vi "CRYCalc Constant Wave Unit.vi"(6 "B_axis mode":u16(slide) scale=0.0..2.0, 7 "A_axis mode":u16(slide) scale=0.0..2.0, 8 "Value in":T2={"Name"="", "Curve"=[], "X data"=1, "Y data"=1, "Z data"=1, "X axis"=0, "Y axis"=1, "Z axis"=1, "X unit"="Hz", "Y unit"="", "Z unit"="deg.", "X dB ref"=1.0, "Y dB ref"=1.0, "Z dB ref"=1.0, "single val"=FALSE, "protected"=FALSE, "display X"=TRUE, "display Y"=TRUE, "display Z"=TRUE, "Test Info"="", "Step No."=0, "Plot Settings"={"Color"=0, "Interpolation"=0, "Point Style"=0, "Line Style"=0, "Point Color"=0, "Line Width"=0, "Bar Plot Style"=0, "Fill To"=0}, "AutoProtect"=FALSE} {"Z data" items=["dB", "Lin"]; "X data" items=["dB", "Lin"]; "Y data" items=["dB", "Lin"]; "Z dB ref" format="%.1f"; "Z axis" items=["Log", "Lin"]; "X dB ref" format="%.1f"; "X axis" items=["Log", "Lin"]; "Y axis" items=["Log", "Lin"]; "Y dB ref" format="%.1f"; "Curve"."z" format="%.2f"; "Curve"."y" format="%.2f"; "Curve"."x" format="%.2f"}, 9 "Work in":u16(slide), 10 "Operator":u16(ring) items=["+", "--", "x", "/"], 11 "Wave in":T1={"Waveform"={"X0"=0.0, "dX"=0.0, "Y"=[]}, "X data"=1, "Y data"=1, "Y axis"=1, "X unit"="s", "Y unit"="V", "Y dB ref"=1.0, "display Y"=TRUE, "display X"=TRUE, "Overload?"=FALSE, "Test Info"="", "Step No."=0, "Name"="", "protected"=FALSE, "Sqc history"=[], "Signal Channel ID"=0, "Plot Settings"={"Color"=0, "Interpolation"=0, "Point Style"=0, "Line Style"=0, "Point Color"=0, "Line Width"=0, "Bar Plot Style"=0, "Fill To"=0}, "AutoProtect"=FALSE} {"Y dB ref" format="%.1f"; "Y axis" items=["Log", "Lin"]; "Y data" items=["dB", "Lin"]; "X data" items=["dB", "Lin"]}) -> (2 "Wave out":T1={"Waveform"={"X0"=0.0, "dX"=0.0, "Y"=[]}, "X data"=1, "Y data"=1, "Y axis"=1, "X unit"="s", "Y unit"="V", "Y dB ref"=1.0, "display Y"=TRUE, "display X"=TRUE, "Overload?"=FALSE, "Test Info"="", "Step No."=0, "Name"="", "protected"=FALSE, "Sqc history"=[], "Signal Channel ID"=0, "Plot Settings"={"Color"=0, "Interpolation"=0, "Point Style"=0, "Line Style"=0, "Point Color"=0, "Line Width"=0, "Bar Plot Style"=0, "Fill To"=0}, "AutoProtect"=FALSE} {"Y dB ref" format="%.1f"; "Y axis" items=["Log", "Lin"]; "Y data" items=["dB", "Lin"]; "X data" items=["dB", "Lin"]})   [LabVIEW 2013]
uses:
  Typedef Control/CRYWaveform Cluster.ctl
  Typedef Control/CRYData Cluster.ctl
  CRYPost Processing Global.vi
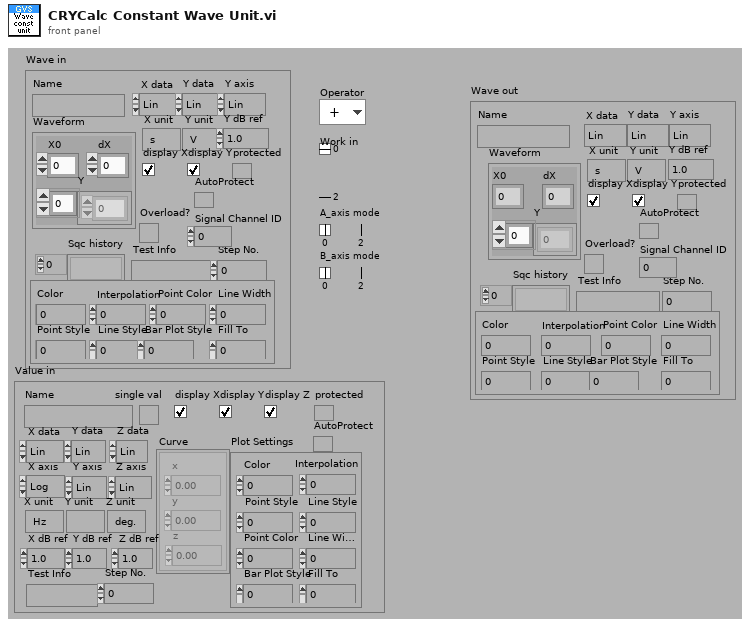
[diagram p1: front panel]
types:
  T1 = typedef "CRYWaveform Cluster.ctl" = cluster{"Waveform":cluster{"X0":dbl, "dX":dbl, "Y":sgl[]}, "X data":u16, "Y data":u16, "Y axis":u16, "X unit":string, "Y unit":string, "Y dB ref":dbl, "display Y":bool, "display X":bool, "Overload?":bool, "Test Info":string, "Step No.":i32, "Name":string, "protected":bool, "Sqc history":string[], "Signal Channel ID":i32, "Plot Settings":cluster{"Color":u32, "Interpolation":u8, "Point Style":u8, "Line Style":u8, "Point Color":u32, "Line Width":u8, "Bar Plot Style":u8, "Fill To":i16}, "AutoProtect":bool}
  T2 = typedef "CRYData Cluster.ctl" = cluster{"Name":string, "Curve":cluster{"x":dbl, "y":dbl, "z":dbl}[], "X data":u16, "Y data":u16, "Z data":u16, "X axis":u16, "Y axis":u16, "Z axis":u16, "X unit":string, "Y unit":string, "Z unit":string, "X dB ref":dbl, "Y dB ref":dbl, "Z dB ref":dbl, "single val":bool, "protected":bool, "display X":bool, "display Y":bool, "display Z":bool, "Test Info":string, "Step No.":i32, "Plot Settings":cluster{"Color":u32, "Interpolation":u8, "Point Style":u8, "Line Style":u8, "Point Color":u32, "Line Width":u8, "Bar Plot Style":u8, "Fill To":i16}, "AutoProtect":bool}
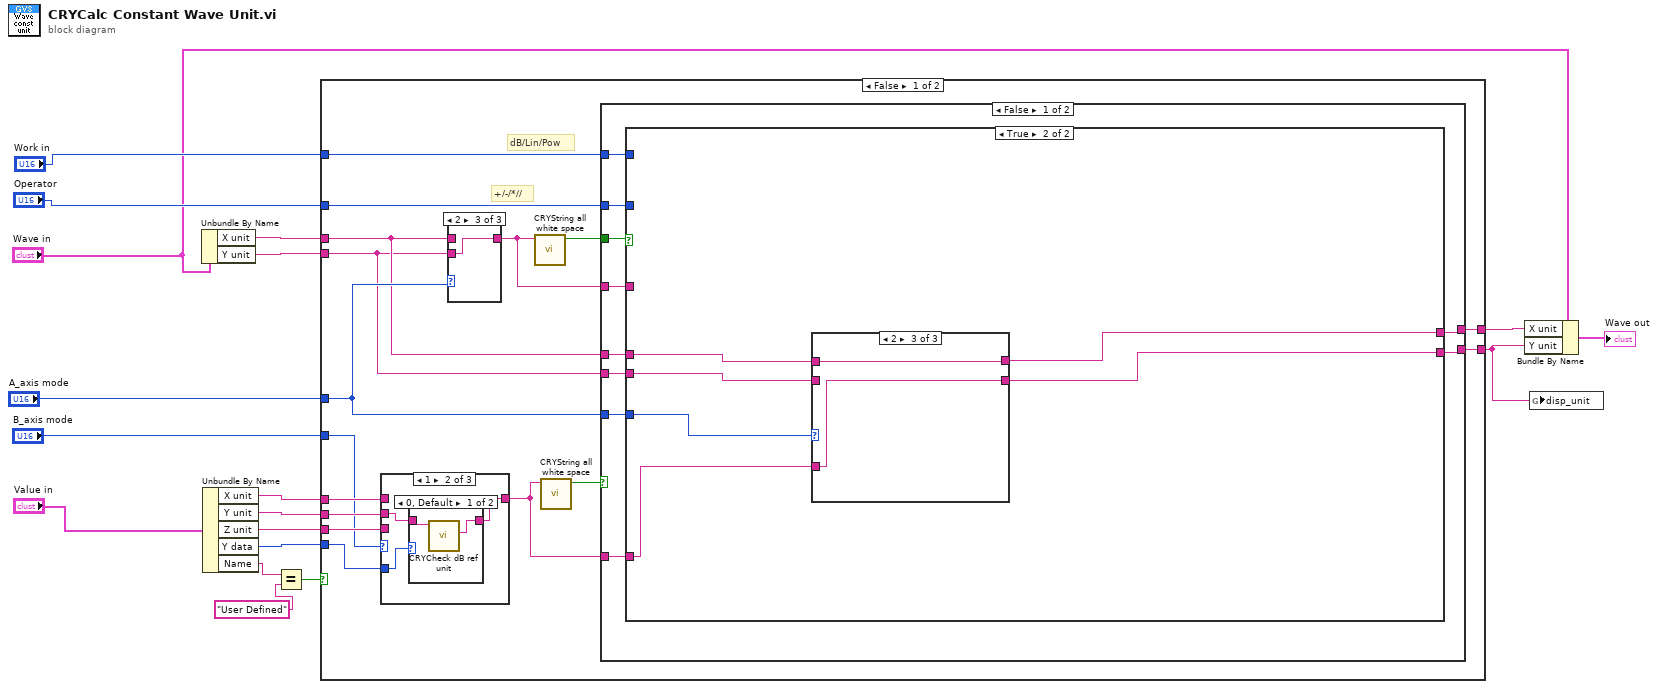
[diagram p0: block diagram]
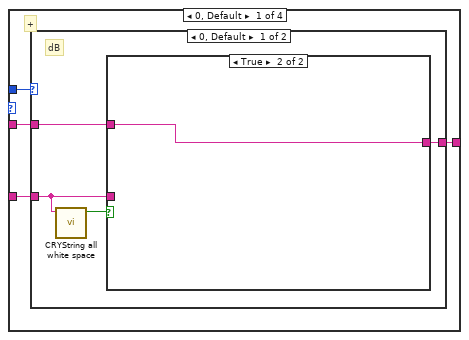
[diagram p7: hidden frame]
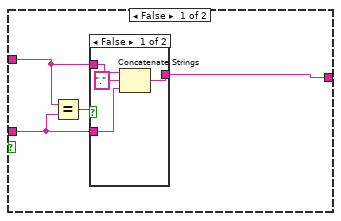
[diagram p8: hidden frame]
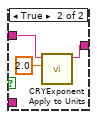
[diagram p9: hidden frame]
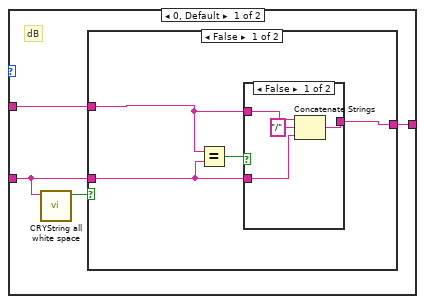
[diagram p11: hidden frame]
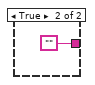
[diagram p12: hidden frame]
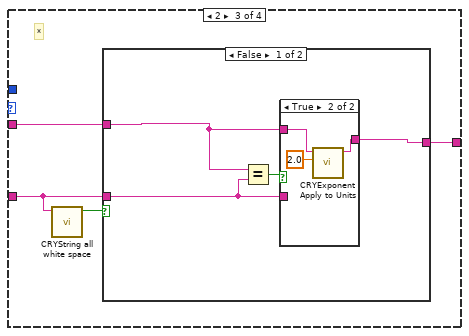
[diagram p14: hidden frame]
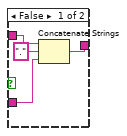
[diagram p15: hidden frame]
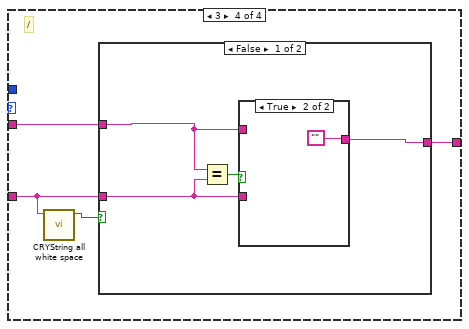
[diagram p17: hidden frame]
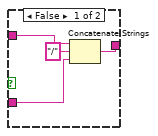
[diagram p18: hidden frame]
diagram:
  n1 = Unbundle By Name("Wave in") -> ("X unit"=w17:string, "Y unit"=w8:string)
  n2 = Unbundle By Name("Value in") -> ("X unit"=w16:string, "Y unit"=w18:string, "Z unit"=w15:string, "Y data"=w10:u16, "Name"=w13:string)
  n3 = Equal?(x=w13, y="User Defined") -> (x = y?=w11:bool)
  n4 = case shown="False" w11 {
    tunnel: w8 -> [w31 w162]
    tunnel: "Operator" -> [w25 _]
    tunnel: "Work in" -> [w26 _]
    tunnel: w18 -> [w23 _]
    tunnel: "A_axis mode" -> [w33 _]
    tunnel: "B_axis mode" -> [w21 _]
    tunnel: w17 -> [w32 w163]
    tunnel: w16 -> [w24 _]
    tunnel: w15 -> [w22 _]
    tunnel: [w29 w163] -> w12
    tunnel: [w30 w162] -> w9
    tunnel: w10 -> [w19 _]
    frame False {
      # "+/-/*//"
      # "dB/Lin/Pow"
      n5 = case shown="1" w21 {
        tunnel: w24 -> [w35 _ _]
        tunnel: w23 -> [_ w37 _]
        tunnel: w22 -> [_ _ w42]
        tunnel: [w35 w36 w42] -> w20
        tunnel: w19 -> [_ w38 _]
        frame 0, Default {
        }
        frame 1 {
          n6 = case shown="0, Default" w38 {
            tunnel: w37 -> [w40 w41]
            tunnel: [w39 w41] -> w36
            frame 0, Default {
              n7 = call "CRYCheck dB ref unit.vi"("Unit in"=w40) -> ("Lin unit out"=w39:string)  [unwired: 1 in, 9 out]
            }
            frame 1 {
            }
          }
        }
        frame 2 {
        }
      }
      n8 = case shown="2" w33 {
        tunnel: w32 -> [w159 w160 _]
        tunnel: w31 -> [_ _ w161]
        tunnel: [w159 w160 w161] -> w27
        frame 0, Default {
        }
        frame 1 {
        }
        frame 2 {
        }
      }
      n9 = call "CRYString all white space.vi"("String"=w27) -> ("Nothing but white space?"=w28:bool)  [unwired: 10 in]
      n10 = call "CRYString all white space.vi"("String"=w20) -> ("Nothing but white space?"=w34:bool)  [unwired: 10 in]
      n11 = case shown="False" w34 {
        tunnel: w33 -> [w52 _]
        tunnel: w32 -> [w49 w158]
        tunnel: w31 -> [w51 w157]
        tunnel: [w50 w157] -> w30
        tunnel: [w47 w158] -> w29
        tunnel: w20 -> [w48 _]
        tunnel: w28 -> [w46 _]
        tunnel: w27 -> [w45 _]
        tunnel: w26 -> [w44 _]
        tunnel: w25 -> [w43 _]
        frame False {
          n12 = case shown="True" w46 {
            tunnel: w52 -> [w53 w150]
            tunnel: w51 -> [w57 w149]
            tunnel: [w55 w148] -> w50
            tunnel: w49 -> [w58 w147]
            tunnel: w48 -> [w59 w146]
            tunnel: [w54 w145] -> w47
            tunnel: w45 -> [w60 _]
            tunnel: w44 -> [w61 _]
            tunnel: w43 -> [w62 _]
            frame False {
              n13 = case shown="2" w53 {
                tunnel: w62 -> [_ w68]
                tunnel: w61 -> [_ w67]
                tunnel: w60 -> [w63 w66]
                tunnel: w59 -> [_ w65]
                tunnel: [w63 w64] -> w56
                frame 0, 1, Default {
                }
                frame 2 {
                  n14 = case shown="1" w68 {
                    tunnel: w67 -> [w72 w93 _ _]
                    tunnel: w66 -> [w71 w92 w112 w128]
                    tunnel: w65 -> [w70 w91 w110 w126]
                    tunnel: [w69 w90 w111 w127] -> w64
                    frame 0, Default {
                      # "+"
                      n15 = case shown="0, Default" w72 {
                        tunnel: w71 -> [w76 w89]
                        tunnel: w70 -> [w74 _]
                        tunnel: [w75 w89] -> w69
                        frame 0, Default {
                          # "dB"
                          n16 = call "CRYString all white space.vi"("String"=w74) -> ("Nothing but white space?"=w73:bool)  [unwired: 10 in]
                          n17 = case shown="True" w73 {
                            tunnel: w76 -> [w80 w88]
                            tunnel: [w79 w88] -> w75
                            tunnel: w74 -> [w78 _]
                            frame False {
                              n18 = Equal?(x=w80, y=w78) -> (x = y?=w77:bool)
                              n19 = case shown="False" w77 {
                                tunnel: w80 -> [w83 w86]
                                tunnel: [w84 w85] -> w79
                                tunnel: w78 -> [w81 _]
                                frame False {
                                n20 = Concatenate Strings(w83, "." ("string"), w81) -> (w84:string)
                                }
                                frame True {
                                n21 = call "CRYExponent Apply to Units.vi"("Exponent to apply"=2.0, "Unit in"=w86) -> ("Unit out"=w85:string)  [unwired: 9 out]
                                }
                              }
                            }
                            frame True {
                            }
                          }
                        }
                        frame 1, 2 {
                          # "Lin,Pow"
                        }
                      }
                    }
                    frame 1 {
                      # "-"
                      n22 = case shown="1, 2" w93 {
                        tunnel: w92 -> [w97 w108]
                        tunnel: w91 -> [w95 _]
                        tunnel: [w96 w108] -> w90
                        frame 0, Default {
                          # "dB"
                          n23 = call "CRYString all white space.vi"("String"=w95) -> ("Nothing but white space?"=w94:bool)  [unwired: 10 in]
                          n24 = case shown="False" w94 {
                            tunnel: w97 -> [w101 w107]
                            tunnel: [w100 w107] -> w96
                            tunnel: w95 -> [w99 _]
                            frame False {
                              n25 = Equal?(x=w101, y=w99) -> (x = y?=w98:bool)
                              n26 = case shown="False" w98 {
                                tunnel: w101 -> [w104 _]
                                tunnel: [w105 ""] -> w100
                                tunnel: w99 -> [w102 _]
                                frame False {
                                n27 = Concatenate Strings(w104, "/" ("string"), w102) -> (w105:string)
                                }
                                frame True {
                                }
                              }
                            }
                            frame True {
                            }
                          }
                        }
                        frame 1, 2 {
                          # "Lin,Pow"
                        }
                      }
                    }
                    frame 2 {
                      # "*"
                      n28 = call "CRYString all white space.vi"("String"=w110) -> ("Nothing but white space?"=w109:bool)  [unwired: 10 in]
                      n29 = case shown="False" w109 {
                        tunnel: w112 -> [w116 w124]
                        tunnel: [w115 w124] -> w111
                        tunnel: w110 -> [w114 _]
                        frame False {
                          n30 = Equal?(x=w116, y=w114) -> (x = y?=w113:bool)
                          n31 = case shown="True" w113 {
                            tunnel: w116 -> [w119 w122]
                            tunnel: [w120 w121] -> w115
                            tunnel: w114 -> [w117 _]
                            frame False {
                              n32 = Concatenate Strings(w119, "." ("string"), w117) -> (w120:string)
                            }
                            frame True {
                              n33 = call "CRYExponent Apply to Units.vi"("Exponent to apply"=2.0, "Unit in"=w122) -> ("Unit out"=w121:string)  [unwired: 9 out]
                            }
                          }
                        }
                        frame True {
                        }
                      }
                    }
                    frame 3 {
                      # "/"
                      n34 = call "CRYString all white space.vi"("String"=w126) -> ("Nothing but white space?"=w125:bool)  [unwired: 10 in]
                      n35 = case shown="False" w125 {
                        tunnel: w128 -> [w132 w138]
                        tunnel: [w131 w138] -> w127
                        tunnel: w126 -> [w130 _]
                        frame False {
                          n36 = Equal?(x=w132, y=w130) -> (x = y?=w129:bool)
                          n37 = case shown="True" w129 {
                            tunnel: w132 -> [w135 _]
                            tunnel: [w136 ""] -> w131
                            tunnel: w130 -> [w133 _]
                            frame False {
                              n38 = Concatenate Strings(w135, "/" ("string"), w133) -> (w136:string)
                            }
                            frame True {
                            }
                          }
                        }
                        frame True {
                        }
                      }
                    }
                  }
                }
              }
              n39 = case shown="2" w53 {
                tunnel: w58 -> [w139 w142 w144]
                tunnel: w57 -> [w140 w141 _]
                tunnel: w56 -> [_ _ w143]
                tunnel: [w140 w141 w143] -> w55
                tunnel: [w139 w142 w144] -> w54
                frame 0, Default {
                }
                frame 1 {
                }
                frame 2 {
                }
              }
            }
            frame True {
              n40 = case shown="2" w150 {
                tunnel: w147 -> [w152 w154 w156]
                tunnel: w149 -> [w151 w153 _]
                tunnel: [w151 w153 w155] -> w148
                tunnel: [w152 w154 w156] -> w145
                tunnel: w146 -> [_ _ w155]
                frame 0, Default {
                }
                frame 1 {
                }
                frame 2 {
                }
              }
            }
          }
        }
        frame True {
        }
      }
    }
    frame True {
      # "Constant"
    }
  }
  n41 = Bundle By Name(cluster="Wave in", "X unit"=w12, "Y unit"=w9) -> (→"Wave out":T1)
  n42 = global write "CRYPost Processing Global.vi" "disp_unit"(w9) -> ()
